vi "Edit INI keys.vi"(8 "error in (no error)":errorcluster, 10 "Keys to edit":T1[](array[typedef]), 11 "INI file path":path) -> (0 "error out":errorcluster, 3 "Errors":string[](array[string]))   [LabVIEW 2015, in "RT Management.lvlib"]
doc: "Adds or edits INI keys."
uses:
  RT Management.lvlib
  controls/INI key.ctl
  <vilib>/Utility/config.llb/Write Key (String).vi
  <vilib>/Utility/config.llb/NI_LVConfig.lvlib
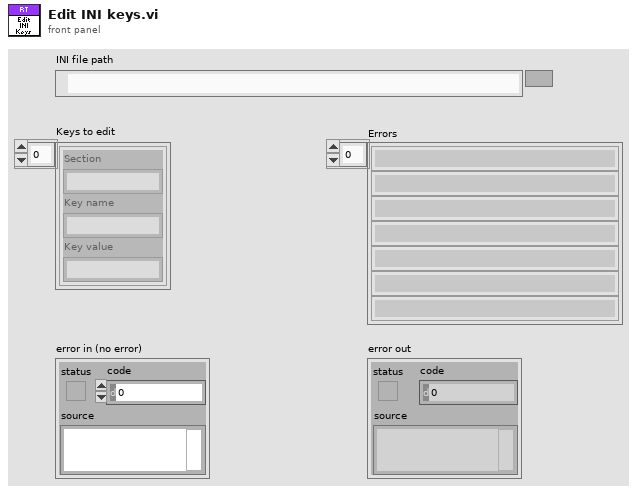
[diagram p1: front panel]
types:
  T1 = typedef "RT Management.lvlib/INI key.ctl" = cluster{"Section":string, "Key name":string, "Key value":string}
  T2 = typedef "NI_LVConfig.lvlib/Config Data RefNum.ctl" = refnum<k1>
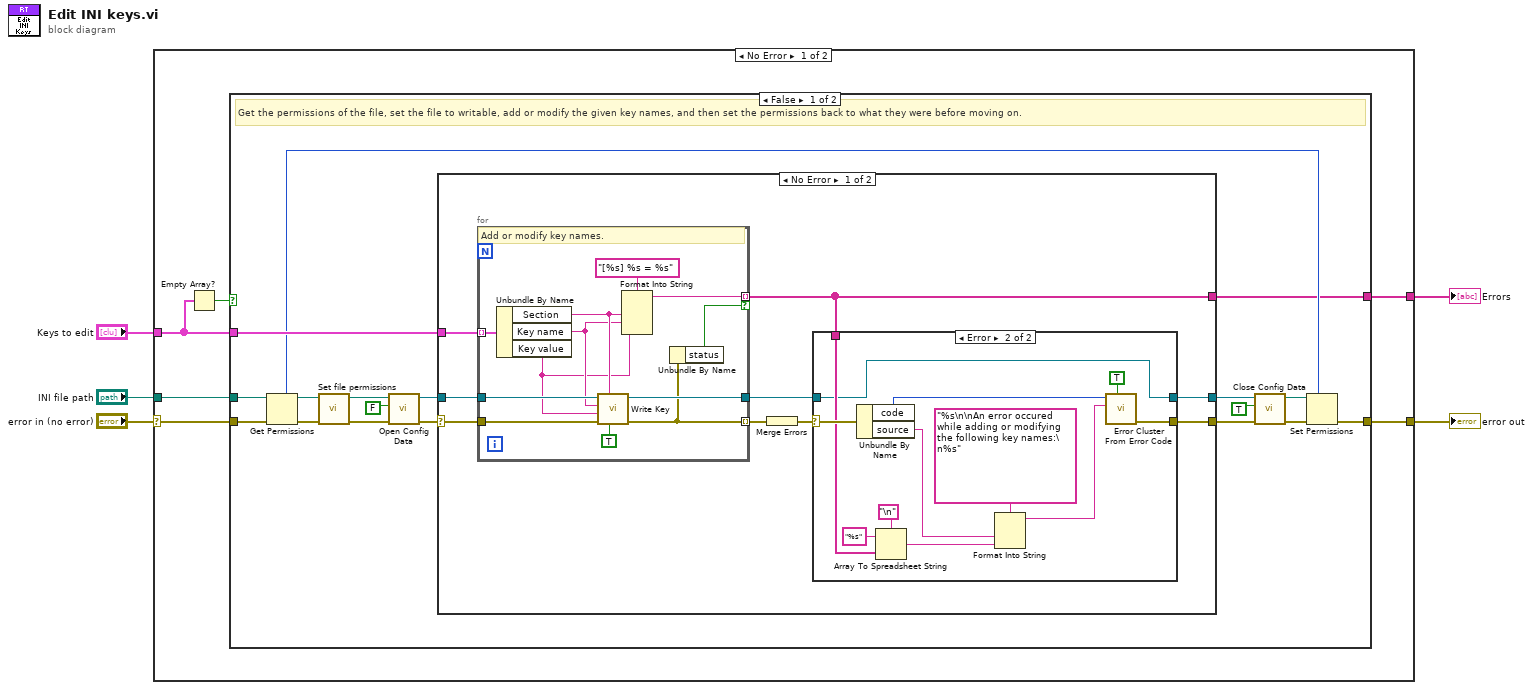
[diagram p0: block diagram]
diagram:
  n1 = case shown="No Error" "error in (no error)" {
    selector: "error in (no error)" -> [w7 w68]
    tunnel: "INI file path" -> [w11 _]
    tunnel: "Keys to edit" -> [w10 _]
    tunnel: [w8 w68] -> w3
    tunnel: [w6 _] -> w1
    frame No Error {
      n2 = Empty Array?(array=w10) -> (empty?=w9:bool)
      n3 = case shown="False" w9 {
        tunnel: w11 -> [w22 _]
        tunnel: w10 -> [w26 _]
        tunnel: [w14 w67] -> w8
        tunnel: w7 -> [w21 w67]
        tunnel: [w12 _] -> w6
        frame False {
          # "Get the permissions of the file, set the file to writable, add or modify the given key names, and then set the permissions back to what they were before moving on."
          n4 = Get Permissions(8:w21, 11:w22) -> (0:w20:errorcluster, 3:w19:path, 5:w13:i16)  [unwired: 2 out]
          n5 = call "Set file permissions.vi"("error in"=w20, "Path"=w19) -> ("error out"=w18:errorcluster, "Path Out"=w17:path)  [unwired: 8 in]
          n6 = call <vilib>:"Open Config Data.vi"("error in (no error)"=w18, "create file if necessary (T)"=FALSE, "configuration file path"=w17) -> ("error out"=w27:errorcluster, "refnum"=w28:T2)  [unwired: 6 in, 1 out]
          n7 = case shown="No Error" w27 {
            selector: w27 -> [w36 w66]
            tunnel: w26 -> [w38 _]
            tunnel: w28 -> [w37 w65]
            tunnel: [w31 w66] -> w24
            tunnel: [w32 w65] -> w25
            tunnel: [w30 _] -> w12
            frame No Error {
              n8 = for {
                tunnel: w38 -> [w62] mode=indexing
                tunnel: w36 -> [w64]
                tunnel: w37 -> [w63]
                tunnel: [w61] -> w33
                tunnel: [w55] -> w35 mode=indexing
                tunnel: [w56] -> w30 mode=indexing if=w54
                # "Add or modify key names."
                n9 = Unbundle By Name(w62) -> ("Section"=w59:string, "Key name"=w58:string, "Key value"=w57:string)
                n10 = call-poly <vilib>:"Write Key.vi"("write raw string? (F)"=TRUE, "section"=w59, "error in (no error)"=w64, "value"=w57, "key"=w58, "refnum"=w63) -> ("error out"=w55:errorcluster, "refnum out"=w61:T2)  [unwired: 3 in, 1 out]
                n11 = Format Into String(format string="[%s] %s = %s", w59, w58, w57) -> (resulting string=w56:string)  [unwired: 2 in, 1 out]
                n12 = Unbundle By Name(w55) -> ("status"=w54:bool)
              }
              n13 = Merge Errors(w35) -> (w34:errorcluster)
              n14 = case shown="Error" w34 {
                selector: w34 -> [w39 w51]
                tunnel: w33 -> [w40 w44]
                tunnel: [w40 w44] -> w32
                tunnel: [w39 w52] -> w31
                tunnel: w30 -> [_ w49]
                frame No Error {
                }
                frame Error {
                  n15 = Unbundle By Name(w51) -> ("code"=w50:i32, "source"=w41:string)
                  n16 = Array To Spreadsheet String(delimiter (Tab)="\n", array=w49, 3:"%s" ("format string")) -> (spreadsheet string=w42:string)
                  n17 = Format Into String(format string="%s\n\nAn error occured while adding or modifying the following key names:\n%s", w41, w42) -> (resulting string=w45:string)  [unwired: 2 in, 1 out]
                  n18 = call <vilib>:"Error Cluster From Error Code.vi"("show call chain? (False)"=TRUE, "error message (\"\")"=w45, "error code (0)"=w50) -> ("error out"=w52:errorcluster)  [unwired: 6 in]
                }
              }
            }
            frame Error {
              # "Something went wrong with getting the file permissions, setting the file to writable, or the file doesn't exist."
            }
          }
          n19 = call <vilib>:"Close Config Data.vi"("error in (no error)"=w24, "write file if changed (T)"=TRUE, "refnum"=w25) -> ("error out"=w16:errorcluster, "file path"=w15:path)  [unwired: 7 in]
          n20 = Set Permissions(7:w13, 8:w16, 11:w15) -> (0:w14:errorcluster)  [unwired: 2 in, 1 out]
        }
        frame True {
          # "The Keys to remove array control is empty."
        }
      }
    }
    frame Error {
    }
  }
  "error out" <- w3
  "Errors" <- w1
